vi "Dequeue.vi"(8 "Error In":errorcluster, 9 "timeout (ms) (Default = -1)":i32=-1) -> (0 "Error Out":errorcluster, 2 "Data":variant, 3 "Command":T1=enum."Close Module")   [LabVIEW 2023, in "Error Manager.lvlib" / "New Error Window.lvlib" / "MHL Queue.lvlib"]
doc: "Receives a command and feeds it to the module Message Handling Loop (MHL)."
uses:
  MHL Queue.lvlib
  Command (enum).ctl
  Queue Reference (library variable).vi
panel:
  # "Input\nInputs to the VI"
  # "Development\nControls or indicators that are useful for development or testing, but which are not outputs of the VI."
  # "Output\nOutputs of the VI"
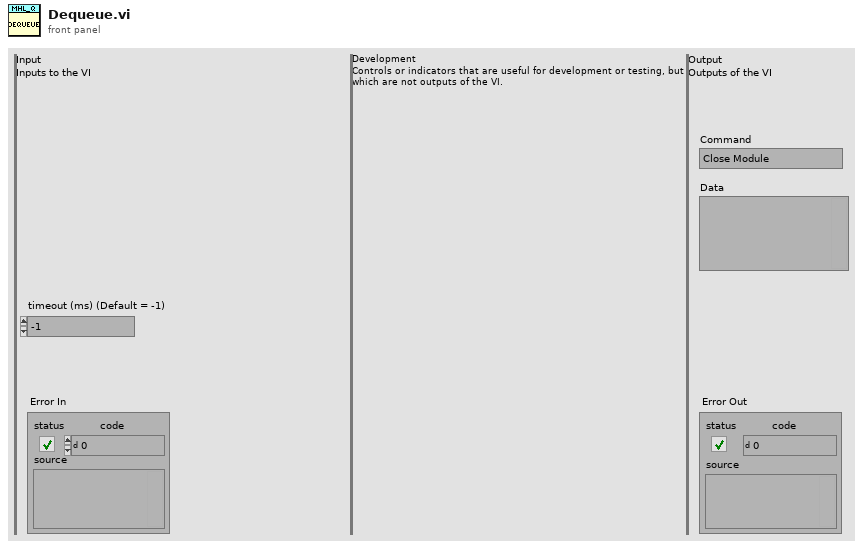
[diagram p1: front panel]
types:
  T1 = typedef "Error Manager.lvlib/New Error Window.lvlib/MHL Queue.lvlib/Command (enum).ctl" = enum16{"Init Module", "Close Module", "Handle Local Error", "OK Button Pressed"}
  T2 = typedef "Error Manager.lvlib/New Error Dialogue GUI.lvlib/MHL Queue.lvlib/Message (cluster).ctl" = cluster{"Command":T3, "Data":variant}
  T3 = typedef "Error Manager.lvlib/New Error Dialogue GUI.lvlib/MHL Queue.lvlib/Command (enum).ctl" = enum16{"Init Module", "Close Module", "Handle Local Error", "OK Button Pressed"}
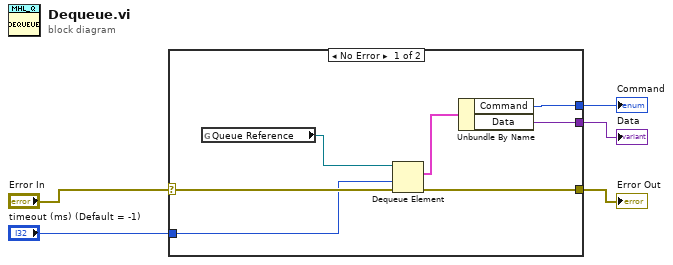
[diagram p0: block diagram]
diagram:
  n1 = case shown="No Error" "Error In" {
    selector: "Error In" -> [w12 w13]
    tunnel: [w11 w13] -> w4
    tunnel: "timeout (ms) (Default = -1)" -> [w10 _]
    tunnel: [w8 _] -> w2
    tunnel: [w7 _] -> w1
    frame No Error {
      n2 = global read "Queue Reference (library variable).vi" "Queue Reference"() -> (w6:refnum<queue>)
      n3 = Dequeue Element(queue=w6, timeout in ms (-1)=w10, error in (no error)=w12) -> (element=w9:T2, error out=w11:errorcluster)  [unwired: 2 out]
      n4 = Unbundle By Name(w9) -> ("Command"=w8:T3, "Data"=w7:variant)
    }
    frame Error {
    }
  }
  "Error Out" <- w4
  "Command" <- w2
  "Data" <- w1
